vi "SpreadsheetTo2Arrays.vi"(5 "file path (dialog if empty)":path) -> (0 "Y Data":dbl[](array[numeric]), 1 "X Data":dbl[](array[numeric]), 2 "EOF?":bool)   [LabVIEW 2017]
doc: "Takes a tab delimited text file and outputs an X array and Y array.\nFirst row can have text or headers\nData should start on the 2nd row."
uses:
  <vilib>/Utility/file.llb/Read Delimited Spreadsheet (DBL).vi
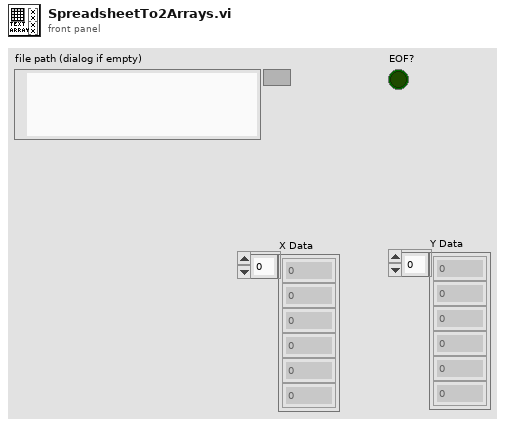
[diagram p1: front panel]
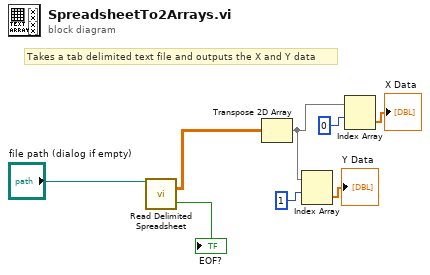
[diagram p0: block diagram]
diagram:
  # "Takes a tab delimited text file and outputs the X and Y data"
  n1 = call-poly <vilib>:"Read Delimited Spreadsheet.vi"("file path (dialog if empty)"="file path (dialog if empty)") -> ("all rows"=w6:dbl[][], "EOF?"=→"EOF?":bool)  [unwired: 9 in, 4 out]
  n2 = Transpose 2D Array(2D array=w6) -> (transposed array=w3:dbl[][])
  n3 = Index Array(array=w3, index (row)=1 ("indexX")) -> (element=→"Y Data":dbl[])  [unwired: 1 in]
  n4 = Index Array(array=w3, index (row)=0 ("indexX")) -> (element=→"X Data":dbl[])  [unwired: 1 in]
